vi "TestVI.vi"() -> ()   [LabVIEW 2012]
uses:
  DeviceEnumXControl.xctl
panel:
  in  "stop":bool
  in  "DeviceEnumXControl":string(xcontrol)
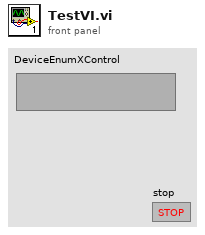
[diagram p1: front panel]
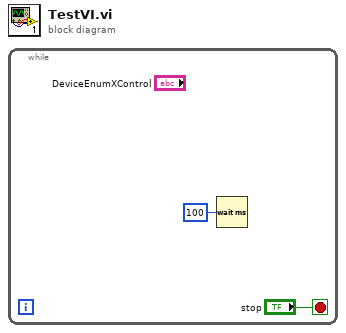
[diagram p0: block diagram]
diagram:
  n1 = while {
    stop <- "stop" stop-if-true
    n2 = Wait (ms)(milliseconds to wait=u32 100) -> ()  [unwired: 1 out]
  }
